vi "udp send test.vi"() -> ()   [LabVIEW 2020]
panel:
  out "error out":errorcluster
  in  "error in":errorcluster
  in  "port or service name":u16=65311
  in  "command in":string="hello"
  in  "Remote Host":string="localhost"
  out "ID fast":refnum<k16>
  in  "timeout ms (100)":i32=100
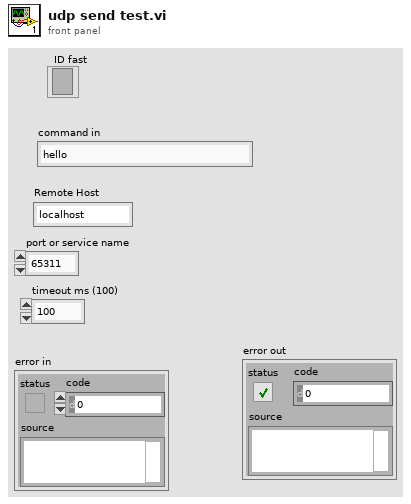
[diagram p1: front panel]
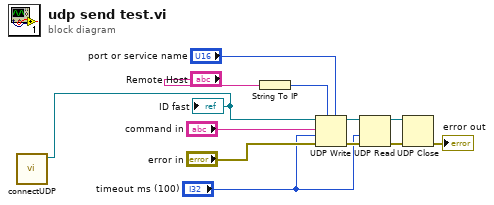
[diagram p0: block diagram]
diagram:
  n1 = call "connectUDP.vi"() -> ("fast ID (h)"=w4:refnum<k16>)  [unwired: 1 in, 3 out]
  "ID fast" <- w4
  n2 = String To IP(1:"Remote Host") -> (0:w7:u32)
  n3 = UDP Write(address=w7, port or service name="port or service name", connection ID=w4, data in="command in", 8:"error in", 9:"timeout ms (100)") -> (error out=w6:errorcluster, 3:w8:refnum<k16>)
  n4 = UDP Read(connection ID=w8, timeout ms (25000)="timeout ms (100)", 8:w6) -> (error out=w3:errorcluster, 3:w2:refnum<k16>)  [unwired: 1 in, 3 out]
  n5 = UDP Close(connection ID=w2, 8:w3) -> (error out=→"error out":errorcluster)  [unwired: 1 out]
